vi "SendMessage.vi"(0 "reference in":refnum<class "TelegramBOT.lvclass">, 2 "sendMessage":T1, 5 "error in (no error)":errorcluster) -> (14 "reference out":refnum<class "TelegramBOT.lvclass">, 19 "error out":errorcluster)   [LabVIEW 2014, in "TelegramBOT.lvclass"]
uses:
  TelegramBOT.lvclass
  SendMessageCluster.ctl
  <vilib>/httpClient/LabVIEWHTTPClient.lvlib
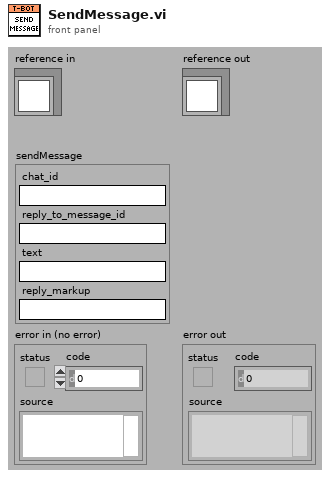
[diagram p1: front panel]
types:
  T1 = typedef "TelegramBOT.lvclass/SendMessageCluster.ctl" = cluster{"chat_id":string, "reply_to_message_id":string, "text":string, "reply_markup":string}
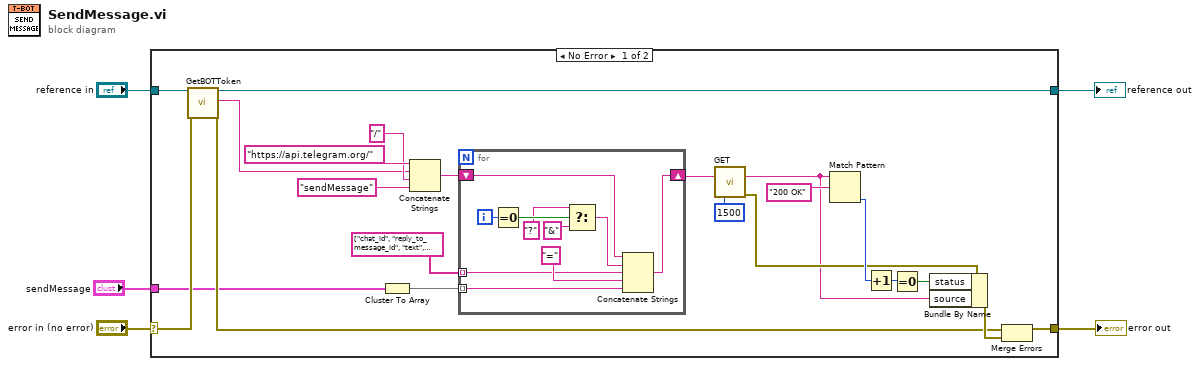
[diagram p0: block diagram]
diagram:
  n1 = case shown="No Error" "error in (no error)" {
    selector: "error in (no error)" -> [w8 w39]
    tunnel: [w7 w39] -> w4
    tunnel: [w9 w38] -> w2
    tunnel: "reference in" -> [w10 w38]
    tunnel: "sendMessage" -> [w6 _]
    frame No Error {
      n2 = call "GetBOTToken.vi"("reference in"=w10, "error in (no error)"=w8) -> ("reference out"=w9:refnum<class "TelegramBOT.lvclass">, "BOTToken"=w15:string, "error out"=w11:errorcluster)  [unwired: 15 in]
      n3 = Cluster To Array(cluster=w6) -> (array=w18:string[])
      n4 = Concatenate Strings("https://api.telegram.org/" ("URL"), w15, "/" ("URL"), "sendMessage" ("URL")) -> (w19:string)
      n5 = for {
        shift-right: [w31] -> w13
        shift-left: w19 -> [w30]
        tunnel: w18 -> [w29] mode=indexing
        tunnel: string[] ["chat_id", "reply_to_message_id", "text", "reply_markup"] ("sendMessageParam") -> [w28] mode=indexing
        i -> [w33]
        n6 = Equal To 0?(x=w33) -> (x = 0?=w36:bool)
        n7 = Select(t="?", s=w36, f="&") -> (s? t:f=w32:string)
        n8 = Concatenate Strings(w30, w32, w28, "=" ("string"), w29) -> (w31:string)
      }
      n9 = call <vilib>:"GET.vi"("url"=w13, "timeout (10000)"=1500) -> ("headers"=w21:string, "error out"=w23:errorcluster)  [unwired: 10 in, 2 out]
      n10 = Match Pattern(string=w21, regular expression="200 OK") -> (offset past match=w25:i32)  [unwired: 1 in, 3 out]
      n11 = Increment(x=w25) -> (x+1=w24:i32)
      n12 = Equal To 0?(x=w24) -> (x = 0?=w22:bool)
      n13 = Bundle By Name(cluster=w23, "status"=w22, "source"=w21) -> (w12:errorcluster)
      n14 = Merge Errors(w11, w12) -> (w7:errorcluster)
    }
    frame Error {
    }
  }
  "error out" <- w4
  "reference out" <- w2
